vi "Close.vi"(8 "error in (no error)":errorcluster, 11 "Data in":refnum<class "SynchType_CEXT.lvclass">) -> (0 "error out":errorcluster, 3 "Data out":refnum<class "SynchType_CEXT.lvclass">)   [LabVIEW 2021, in "BT.lvlib" / "SynchType_CEXT.lvclass"]
doc: "Abstract Data Classes 2.1.1.12\nTim Streeter - TSA\nCopyright (c) 2024, TSA"
uses:
  SynchType_CEXT.lvclass
  SynchType_CEXT.lvclass/SynchType_CEXT.ctl
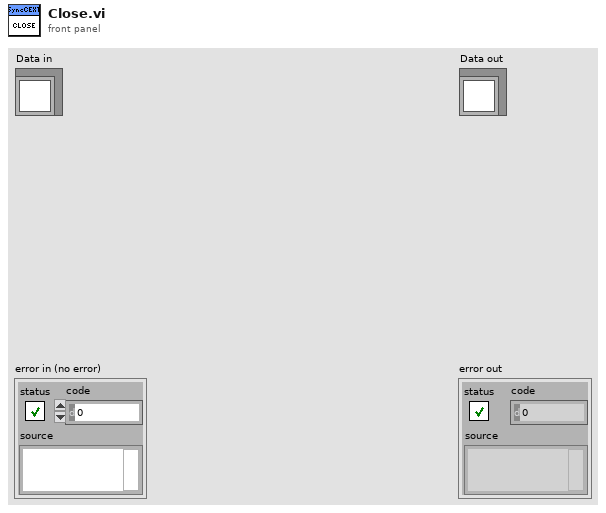
[diagram p1: front panel]
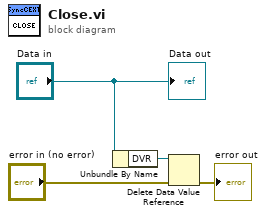
[diagram p0: block diagram]
diagram:
  n1 = Unbundle By Name("Data in") -> ("DVR"=w1:refnum<data-value>)
  n2 = Delete Data Value Reference(data value reference=w1, error in="error in (no error)") -> (error out=→"error out":errorcluster)  [unwired: 1 out]
  "Data out" <- "Data in"
